vi "SimpleReadIG.vi"(2 "Error":errorcluster caption="Fehler (Eingang, kein Fehler)", 3 "Address":u8, 4 "Serial Port":refnum<visa-resource-name>="COM1") -> (0 "Fehler (Ausgang)":errorcluster, 1 "Response (First line)":string)   [LabVIEW 2009]
panel:
  out "Command":string
  out "Full Response":string[](array[string])
  in  "Serial Settings:Flow Control":u16(ring) items=["None", "XON/XOFF", "RTS/CTS", "XON/XOFF & RTS/CTS", "DTR/DSR", "XON/XOFF & DTR/DSR"]
  in  "Serial Settings:Stop Bits":u16(ring)=10 items=["1.0"=10, "1.5"=15, "2.0"=20]
  in  "Serial Settings:Parity":u16(ring) items=["None", "Odd", "Even", "Mark", "Space"]
  in  "Serial Settings:Data Bits":u16=8
  in  "Serial Settings:Baud Rate":u32=9600
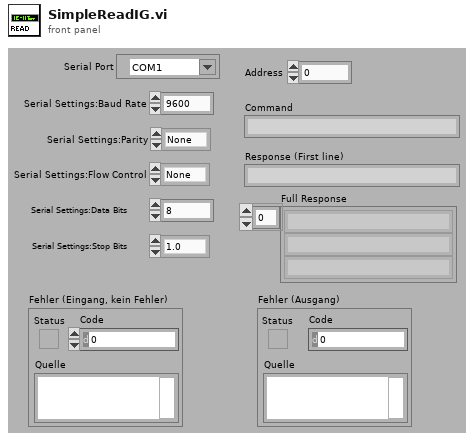
[diagram p1: front panel]
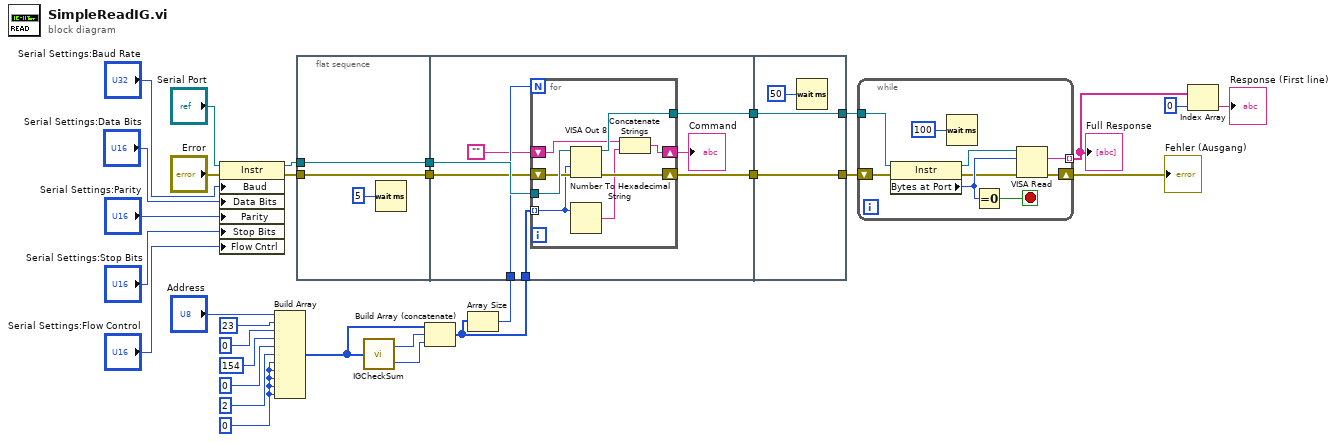
[diagram p0: block diagram]
diagram:
  w25 = u8 0
  n1 = property class="Instr"(reference="Serial Port", error in="Error", "Baud"="Serial Settings:Baud Rate", "Data Bits"="Serial Settings:Data Bits", "Parity"="Serial Settings:Parity", "Stop Bits"="Serial Settings:Stop Bits", "Flow Cntrl"="Serial Settings:Flow Control") -> (reference out=w17:refnum<visa-resource-name>, error out=w14:errorcluster)
  n2 = Build Array("Address", u8 23, u8 0, u8 154, u8 0, u8 2, w25, w25, w25, w25, w25) -> (w24:u8[])
  n3 = flat-sequence {
    tunnel: w14 -> [w33]
    tunnel: w17 -> [w34]
    tunnel: [w34] -> w20
    tunnel: [w33] -> w19
    tunnel: w21 -> [w42]
    tunnel: w20 -> [w41]
    tunnel: w19 -> [w40]
    tunnel: w18 -> [w39]
    tunnel: [w38] -> w8
    tunnel: [w37] -> w7
    tunnel: [w52] -> w2
    tunnel: [w53] -> w1
    tunnel: w8 -> [w53]
    tunnel: w7 -> [w52]
    frame #0 {
      n4 = Wait (ms)(milliseconds to wait=u32 5 ("Zu wartende ms")) -> ()  [unwired: 1 out]
    }
    frame #1 {
      n5 = for {
        N: w39 -> [_]
        tunnel: w42 -> [w43] mode=indexing
        tunnel: w41 -> [w50]
        shift-right: [w48] -> w38
        shift-left: w40 -> [w49]
        tunnel: [w47] -> w37
        shift-right: [w45] -> w35
        shift-left: "" -> [w46]
        n6 = VISA Out 8(8:w49, 9:w43, 11:w50) -> (0:w48:errorcluster, 3:w47:refnum<visa-resource-name>)  [unwired: 2 in]
        n7 = Number To Hexadecimal String(2:w43) -> (0:w44:string)  [unwired: 1 in]
        n8 = Concatenate Strings(w46, w44) -> (w45:string)
      }
      "Command" <- w35
    }
    frame #2 {
      n9 = Wait (ms)(milliseconds to wait=u32 50 ("Zu wartende ms")) -> ()  [unwired: 1 out]
    }
  }
  n10 = call "IGCheckSum.vi"("Input array"=w24) -> ("CRC1"=w23:u8, "CRC0"=w22:u8)
  n11 = Build Array (concatenate)(w24, w23, w22) -> (w21:u8[])
  n12 = Array Size(array=w21) -> (size(s)=w18:i32)
  n13 = while {
    shift-right: [w57] -> w6
    shift-left: w1 -> [w61]
    tunnel: [w56] -> w5 mode=indexing
    tunnel: w2 -> [w54]
    stop <- w62 stop-if-true
    n14 = property class="Instr"(reference=w54, error in=w61) -> (reference out=w60:refnum<visa-resource-name>, error out=w58:errorcluster, "Bytes at Port"=w59:u32)
    n15 = Wait (ms)(milliseconds to wait=u32 100 ("Zu wartende ms")) -> ()  [unwired: 1 out]
    n16 = Equal To 0?(x=w59) -> (x = 0?=w62:bool)
    n17 = VISA Read(VISA resource name=w60, byte count=w59, error in (no error)=w58) -> (read buffer=w56:string, error out=w57:errorcluster)  [unwired: 2 out]
  }
  "Fehler (Ausgang)" <- w6
  "Full Response" <- w5
  n18 = Index Array(array=w5, index=0 ("Index")) -> (element=→"Response (First line)":string)
